vi "Set Segments.vi"(0 "instrument handle":refnum<k15>, 1 "Channel":string, 2 "PowerValues":dbl[](array[numeric])=[10.0] format="%.2p", 3 "NumberPoints":i32[](array[numeric])=[1], 4 "StartFrequency":dbl[](array[numeric])=[1000000000.0] format="%.2p", 5 "StopFrequency":dbl[](array[numeric])=[3000000000.0] format="%.2p", 6 "IFBandWidth":dbl[](array[numeric])=[0.0] format="%.2p", 7 "error in (no error)":errorcluster {"code" format="%.0x"}, 8 "DwellTime":dbl[](array[numeric])=[0.0] format="%.2p") -> (20 "instrument handle out":refnum<k15>, 27 "error out":errorcluster {"code" format="%.0x"})   [LabVIEW 2014, in "Agilent NA.lvlib"]
doc: "Set the entire list of values in the segment sweep table. The first three data elements must always be supplied. After those values, data must be supplied for successive optional elements. For example, to set dwell time values, you must also supply IFBW values, because IFBW (#5) precedes dwell time (#6) in the array order."
uses:
  Agilent NA.lvlib
  AgNA.dll
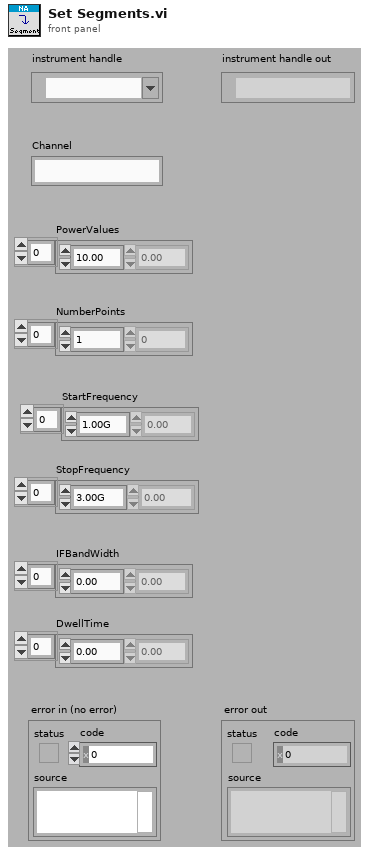
[diagram p1: front panel]
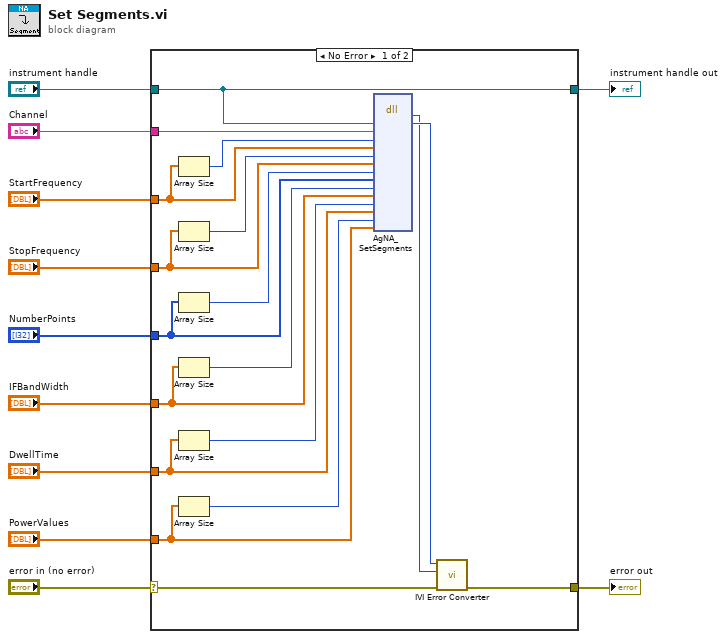
[diagram p0: block diagram]
diagram:
  n1 = case shown="No Error" "error in (no error)" {
    selector: "error in (no error)" -> [w27 w31]
    tunnel: [w26 w31] -> w11
    tunnel: "Channel" -> [w25 _]
    tunnel: "StartFrequency" -> [w22 _]
    tunnel: "StopFrequency" -> [w20 _]
    tunnel: "NumberPoints" -> [w18 _]
    tunnel: "IFBandWidth" -> [w16 _]
    tunnel: "DwellTime" -> [w14 _]
    tunnel: "PowerValues" -> [w12 _]
    tunnel: [w24 w30] -> w2
    tunnel: "instrument handle" -> [w24 w30]
    frame No Error {
      n2 = Array Size(array=w22) -> (size(s)=w23:i32)
      n3 = Array Size(array=w20) -> (size(s)=w21:i32)
      n4 = Array Size(array=w18) -> (size(s)=w19:i32)
      n5 = Array Size(array=w16) -> (size(s)=w17:i32)
      n6 = Array Size(array=w14) -> (size(s)=w15:i32)
      n7 = Array Size(array=w12) -> (size(s)=w13:i32)
      n8 = dll-call lib="AgNA**.dll" fn="AgNA_SetSegments"("Vi"=w24, "Channel"=w25, "StartFrequencyBufferSize"=w23, "StartFrequency"=w22, "StopFrequencyBufferSize"=w21, "StopFrequency"=w20, "NumberPointsBufferSize"=w19, "NumberPoints"=w18, "IFBandWidthBufferSize"=w17, "IFBandWidth"=w16, "DwellTimeBufferSize"=w15, "DwellTime"=w14, "PowerValuesBufferSize"=w13, "PowerValues"=w12) -> (w28:i32, "Vi"=w29:u32)  [unwired: 16 in, 2 out]
      n9 = call "IVI Error Converter.vi"("error in (no error)"=w27, "IVI error code (0)"=w28, "instrument handle"=w29) -> ("error out"=w26:errorcluster)  [unwired: 7 in, 1 out]
    }
    frame Error {
    }
  }
  "error out" <- w11
  "instrument handle out" <- w2
